vi "find_fiducial.vi"(8 "error in":errorcluster, 9 "interactive":bool, 10 "Fiducial Parameters":T1, 11 "Image":T2) -> (0 "error out":errorcluster, 2 "coords":cluster{"x":dbl, "y":dbl}[](array[cluster]))   [LabVIEW 2011, in "gVision.lvlib"]
uses:
  gVision.lvlib
  <vilib>/vision/Image Controls.llb/IMAQ Image.ctl
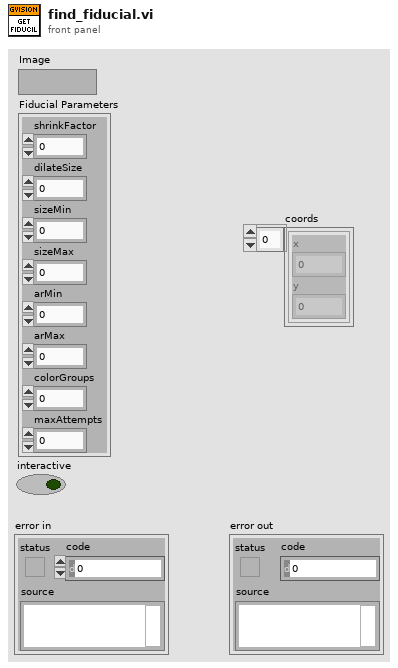
[diagram p1: front panel]
types:
  T1 = cluster{"shrinkFactor":sgl, "dilateSize":i32, "sizeMin":sgl, "sizeMax":sgl, "arMin":sgl, "arMax":sgl, "colorGroups":i32, "maxAttempts":i32}
  T2 = typedef "IMAQ Image.ctl" = refnum<image>
  T3 = enum32{"Map Pixel Pointer", "Unmap Pixel Pointer", "Get Pixels Infos"}
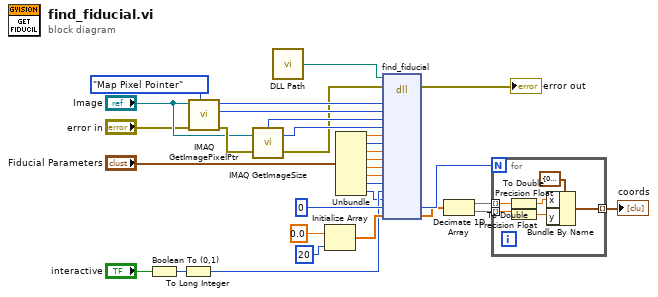
[diagram p0: block diagram]
diagram:
  n1 = Boolean To (0,1)(Boolean="interactive") -> (0, 1=w9:i16)
  n2 = To Long Integer(number=w9) -> (32bit integer=w8:i32)
  n3 = call "IMAQ GetImagePixelPtr"("Function"=T3."Map Pixel Pointer", "error in (no error)"="error in", "Image"="Image") -> ("error out"=w18:errorcluster, "LineWidth(Pixels)"=w15:i32, "Pixel Pointer out"=w16:u64)  [unwired: 3 in, 3 out]
  n4 = call "IMAQ GetImageSize"("Image"="Image", "error in (no error)"=w18) -> ("Y Resolution"=w13:i32, "X Resolution"=w14:i32, "error out"=w11:errorcluster)  [unwired: 2 in]
  n5 = call "DLL Path.vi"() -> ("DLL Path"=w20:path)  [unwired: 5 in]
  n6 = Initialize Array(0.0 ("element"), 20 ("dimension size")) -> (w29:dbl[])
  n7 = Unbundle("Fiducial Parameters") -> ("shrinkFactor"=w27:sgl, "dilateSize"=w21:i32, "sizeMin"=w22:sgl, "sizeMax"=w23:sgl, "arMin"=w24:sgl, "arMax"=w25:sgl, "colorGroups"=w26:i32, "maxAttempts"=w1:i32)
  n8 = dll-call lib="?" fn="find_fiducial"(path in=w20, error in=w11, "imgPtr"=w16, "imgLineWidth"=w15, "imgWidth"=w14, "imgHeight"=w13, "shrinkFactor"=w27, "dilateSize"=w21, "sizeMin"=w22, "sizeMax"=w23, "arMin"=w24, "arMax"=w25, "colorGroups"=w26, "interactive"=w8, "numAttempts"=w1, "numFiducials"=0, "coords"=w29) -> (error out=→"error out":errorcluster, "numFiducials"=w7:i32, "coords"=w6:sgl[])  [unwired: 15 in, 1 out]
  n9 = Decimate 1D Array(w6) -> (w5:sgl[], w4:sgl[])
  n10 = for {
    N: w7 -> [_]
    tunnel: w5 -> [w36] mode=indexing
    tunnel: w4 -> [w35] mode=indexing
    tunnel: [w37] -> w3 mode=indexing
    n11 = To Double Precision Float(number=w36) -> (double precision float=w34:dbl)
    n12 = To Double Precision Float(number=w35) -> (double precision float=w33:dbl)
    n13 = Bundle By Name(cluster=cluster{"x":dbl, "y":dbl} {"x"=0.0, "y"=0.0}, "x"=w34, "y"=w33) -> (w37:cluster{"x":dbl, "y":dbl})
  }
  "coords" <- w3
